vi "Set Random Tracks.vi"(10 "areas":i32, 11 "numTracks":i32) -> (2 "areas out":i32, 3 "function return":u32)   [LabVIEW 2018, in "AndorSDK.lvlib"]
doc: "EXPNETTYPE unsigned int WINAPI SetRandomTracks(int numTracks, int * areas);"
uses:
  AndorSDK.lvlib
  ATMCD32D.dll
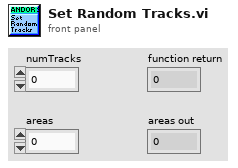
[diagram p1: front panel]
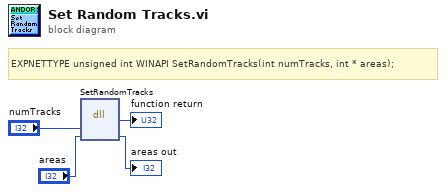
[diagram p0: block diagram]
diagram:
  # "EXPNETTYPE unsigned int WINAPI SetRandomTracks(int numTracks, int * areas);"
  n1 = dll-call lib="PTH2babs E\nPersönliches02 - Arbeit03-HiwijobsLabviewCodelibANDOR\tAndor SDK\nATMCD32D.*" fn="SetRandomTracks"("numTracks"="numTracks", "areas"="areas") -> (→"function return":u32, "areas"=→"areas out":i32)  [unwired: 4 in, 2 out]
